vi "D-Pad Val To Enum.vi"(10 "D-Pad Value":i32) -> (2 "D-Pad Enum":T1)   [LabVIEW 2011, in "LVH-Xbox-One-Controller.lvlib"]
uses:
  LVH-Xbox-One-Controller.lvlib
  Type Defs/Indicators/DPad Enum.ctl
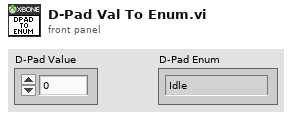
[diagram p1: front panel]
types:
  T1 = typedef "LVH-Xbox-One-Controller.lvlib/DPad Enum.ctl" = enum16{"Idle", "Up", "Up / Right", "Right", "Down / Right", "Down", "Down / Left", "Left", "Up / Left"}
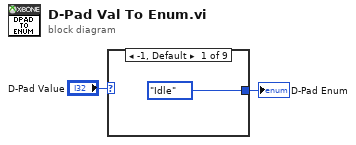
[diagram p0: block diagram]
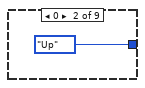
[diagram p2: hidden frame]
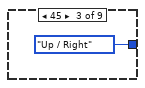
[diagram p3: hidden frame]
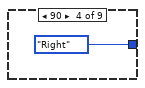
[diagram p4: hidden frame]
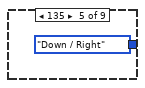
[diagram p5: hidden frame]
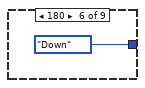
[diagram p6: hidden frame]
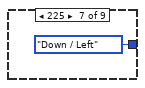
[diagram p7: hidden frame]
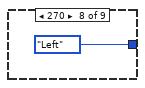
[diagram p8: hidden frame]
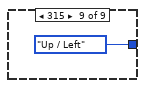
[diagram p9: hidden frame]
diagram:
  n1 = case shown="-1, Default" "D-Pad Value" {
    tunnel: [DPad_Enum."Idle" ("D-Pad") DPad_Enum."Up" ("D-Pad") DPad_Enum."Up / Right" ("D-Pad") DPad_Enum."Right" ("D-Pad") DPad_Enum."Down / Right" ("D-Pad") DPad_Enum."Down" ("D-Pad") DPad_Enum."Down / Left" ("D-Pad") DPad_Enum."Left" ("D-Pad") DPad_Enum."Up / Left" ("D-Pad")] -> w1
    frame -1, Default {
    }
    frame 0 {
    }
    frame 45 {
    }
    frame 90 {
    }
    frame 135 {
    }
    frame 180 {
    }
    frame 225 {
    }
    frame 270 {
    }
    frame 315 {
    }
  }
  "D-Pad Enum" <- w1
